vi "SENS_SWE_DWEL_AUTO_ON_OFF.vi"(0 "VISA IN":refnum<visa-resource-name>, 1 "Dwell ON/OFF":bool, 5 "error in":errorcluster, 7 "Channel":i32) -> (14 "VISA Out":refnum<visa-resource-name>, 19 "error out":errorcluster)   [LabVIEW 2018, in "PNA-X.lvlib"]
doc: "SENSe<cnum>:SWEep:DWELl:AUTO <ON | OFF> \n(Read-Write) Specifies whether or not to automatically calculate and set the minimum possible dwell time. Setting \nAuto ON has the same effect as setting dwell time to 0. \nParameters \n<cnum> Any existing channel number. If unspecified, value is set to 1 \n<ON | OFF> ON (or 1) - turns dwell ON. \nOFF (or 0) - turns dwell OFF. \nExamples SENS:SWE:DWEL:AUTO ON \nsense2:sweep:dwell:auto off \nQuery Syntax SENSe<cnum>:SWEep:DWELl:AUTO? \nReturn Type Boolean (1 = ON, 0 = OFF) \nDefault ON"
uses:
  PNA-X.lvlib
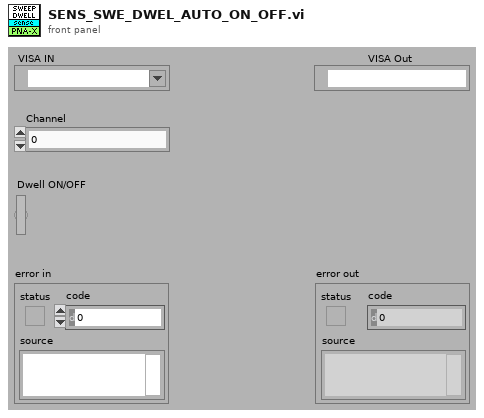
[diagram p1: front panel]
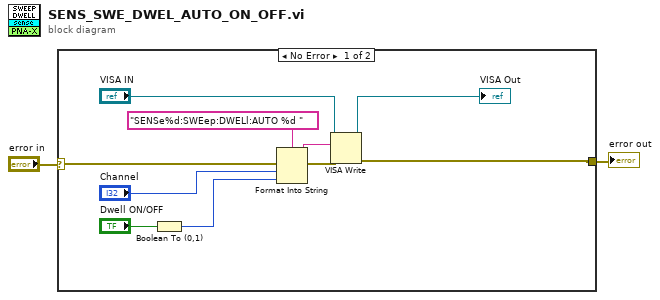
[diagram p0: block diagram]
diagram:
  n1 = case shown="No Error" "error in" {
    selector: "error in" -> [w12 w13]
    tunnel: [w7 w13] -> w1
    frame No Error {
      n2 = Boolean To (0,1)(Boolean="Dwell ON/OFF") -> (0, 1=w3:i16)
      n3 = Format Into String(format string="SENSe%d:SWEep:DWELl:AUTO %d " ("Cmdline"), error in=w12, "Channel", w3) -> (resulting string=w10:string, error out=w11:errorcluster)  [unwired: 1 in]
      n4 = VISA Write(VISA resource name="VISA IN", write buffer=w10, error in (no error)=w11) -> (VISA resource name out=→"VISA Out":refnum<visa-resource-name>, error out=w7:errorcluster)  [unwired: 1 out]
    }
    frame Error {
    }
  }
  "error out" <- w1
